vi "open3000.vi"(4 "ViInfo":T1, 7 "InterfaceInfo":T2) -> (0 "ViInfoOut":T1, 1 "ModuleInfo":T4 {"DacScaleCoef" format="%#_2g"; "DacOffsetCoef" format="%#_2g"}, 3 "InterfaceInfoOut":T2)   [LabVIEW 2010]
panel:
  out "Array":T3(array[ring])
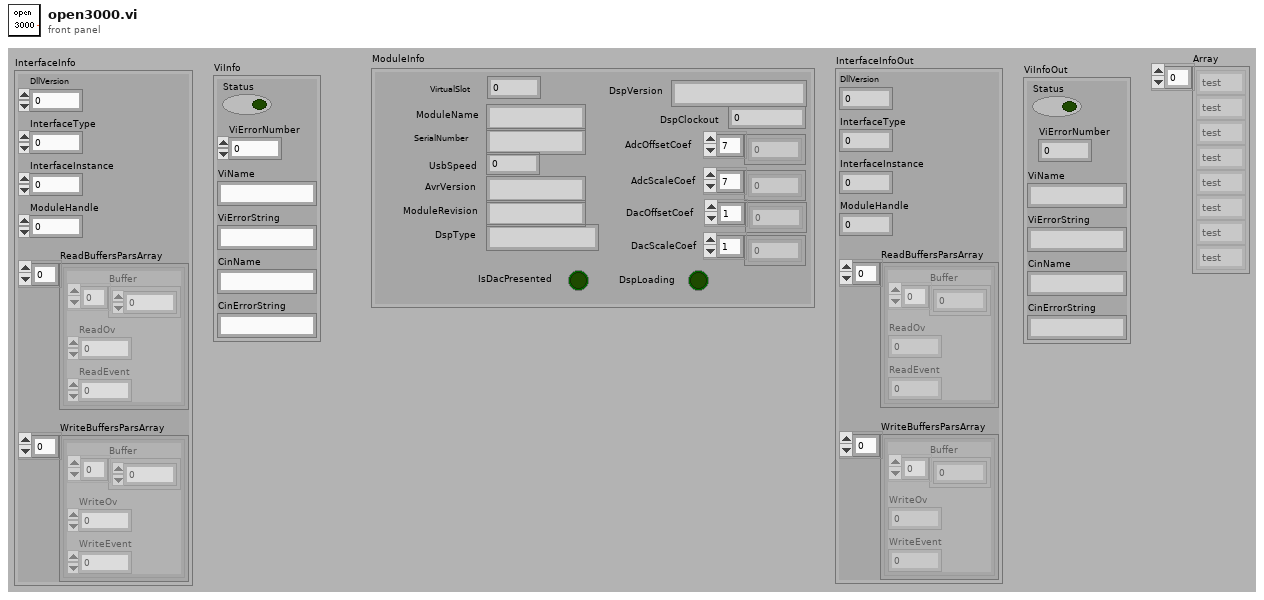
[diagram p1: front panel]
types:
  T1 = cluster{"Status":bool, "ViErrorNumber":u32, "ViName":string, "ViErrorString":string, "CinName":string, "CinErrorString":string}
  T2 = cluster{"DllVersion":u32, "InterfaceType":u32, "InterfaceInstance":u32, "ModuleHandle":u32, "ReadBuffersParsArray":cluster{"Buffer":i16[], "ReadOv":u32, "ReadEvent":u32}[], "WriteBuffersParsArray":cluster{"Buffer":i16[], "WriteOv":u32, "WriteEvent":u32}[]}
  T3 = enum16{"test", "get_slot", "load", "start", "finish", "restart"}[]
  T4 = cluster{"VirtualSlot":u16, "ModuleName":string, "SerialNumber":string, "UsbSpeed":u8, "AvrVersion":string, "ModuleRevision":string, "DspType":string, "IsDacPresented":bool, "DspLoading":bool, "DspVersion":string, "DspClockout":u32, "AdcOffsetCoef":sgl[], "AdcScaleCoef":sgl[], "DacOffsetCoef":sgl[], "DacScaleCoef":sgl[]}
  T5 = enum16{"test", "get_slot", "load", "start", "finish"}
  T6 = enum16{"test", "get_slot", "load", "start", "finish", "restart"}
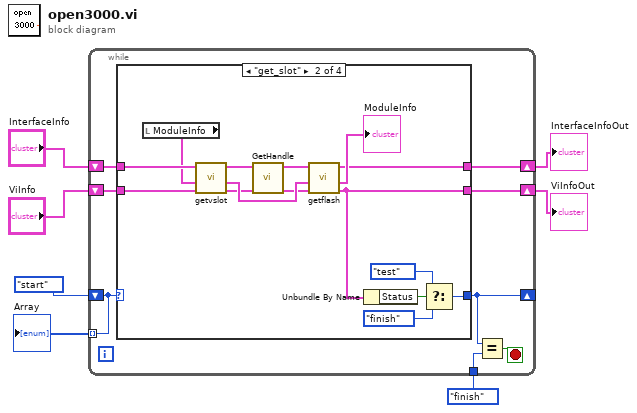
[diagram p0: block diagram]
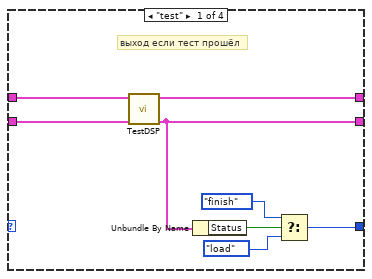
[diagram p2: hidden frame]
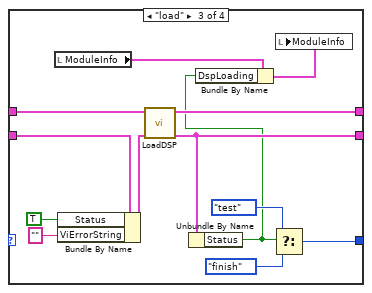
[diagram p3: hidden frame]
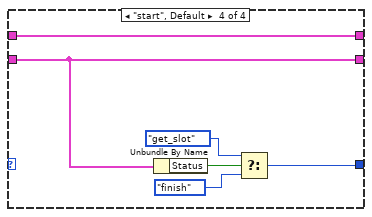
[diagram p4: hidden frame]
diagram:
  n1 = while {
    shift-right: [w14] -> w3
    shift-left: "InterfaceInfo" -> [w15]
    shift-right: [w12] -> w5
    shift-left: "ViInfo" -> [w13]
    shift-right: [w11] -> _
    shift-left: T6."start" -> [w8]
    tunnel: T5."finish" -> [w9]
    tunnel: [w8] -> w7 mode=indexing
    stop <- w10 stop-if-true
    n2 = case shown="\"get_slot\"" w8 {
      tunnel: w15 -> [w23 w32 w51 w57]
      tunnel: [w20 w31 w50 w57] -> w14
      tunnel: w13 -> [w22 w30 w44 w56]
      tunnel: [w17 w26 w49 w56] -> w12
      tunnel: [w18 w27 w47 w52] -> w11
      frame "test" {
        # "выход если тест прошёл"
        n3 = call "TestDSP.vi"("ViInfo"=w22, "InterfaceInfo"=w23) -> ("ViInfoOut"=w17:T1, "InterfaceInfoOut"=w20:T2)  [unwired: 4 in]
        n4 = Unbundle By Name(w17) -> ("Status"=w21:bool)
        n5 = Select(t=T5."finish", s=w21, f=T5."load") -> (s? t:f=w18:T5)
      }
      frame "get_slot" {
        n6 = local read "ModuleInfo"() -> (w24:T4)
        n7 = call "getvslot.vi"("ViInfo"=w30, "ModuleInfoIn"=w24, "InterfaceInfo"=w32) -> ("ViInfoOut"=w35:T1, "ModuleInfo"=w38:T4, "InterfaceInfoOut"=w34:T2)  [unwired: 2 in]
        n8 = call "GetHandle.vi"("Cluster"=w35, "InterfaceInfoIn"=w34) -> ("ClusterOut"=w37:T1, "InterfaceInfo"=w36:T2)  [unwired: 4 in]
        n9 = call "getflash.vi"("ViInfo"=w37, "ModuleInfo"=w38, "InterfaceInfo"=w36) -> ("ViInfo2"=w26:T1, "ModuleInfo 2"=→"ModuleInfo":T4, "InterfaceInfo 2"=w31:T2)  [unwired: 2 in]
        n10 = Unbundle By Name(w26) -> ("Status"=w29:bool)
        n11 = Select(t=T5."test", s=w29, f=T5."finish") -> (s? t:f=w27:T5)
      }
      frame "load" {
        n12 = local read "ModuleInfo"() -> (w41:T4)
        n13 = Bundle By Name(cluster=w44, "Status"=TRUE, "ViErrorString"="") -> (w43:T1)
        n14 = call "LoadDSP.vi"("ViInfo"=w43, "InterfaceInfo"=w51) -> ("ViInfoOut"=w49:T1, "InterfaceInfoOut"=w50:T2)  [unwired: 4 in]
        n15 = Unbundle By Name(w49) -> ("Status"=w45:bool)
        n16 = Bundle By Name(cluster=w41, "DspLoading"=w45) -> (w40:T4)
        n17 = Select(t=T5."test", s=w45, f=T5."finish") -> (s? t:f=w47:T5)
        n18 = local write "ModuleInfo"(w40) -> ()
      }
      frame "start", Default {
        n19 = Unbundle By Name(w56) -> ("Status"=w55:bool)
        n20 = Select(t=T5."get_slot", s=w55, f=T5."finish") -> (s? t:f=w52:T5)
      }
    }
    n21 = Equal?(x=w11, y=w9) -> (x = y?=w10:bool)
  }
  "Array" <- w7
  "ViInfoOut" <- w5
  "InterfaceInfoOut" <- w3
